vi "oa_Full Spectrum Transform (Spectra).vi"(6 "direction":u16(ring)=1 items=["CCW", "CW"], 7 "shift reverse spectrum (T)":bool=TRUE, 9 "phase lag spectrum (X-Y)":cluster{"x0":dbl, "dx":dbl, "phase":dbl[]}, 10 "Y magnitude spectrum":cluster{"x0":dbl, "dx":dbl, "magnitude":dbl[]}, 11 "X magnitude spectrum":cluster{"x0":dbl, "dx":dbl, "magnitude":dbl[]}) -> (2 "reverse precession spectrum":cluster{"x0":dbl, "dx":dbl, "magnitude":dbl[]}, 3 "forward precession spectrum":cluster{"x0":dbl, "dx":dbl, "magnitude":dbl[]})   [LabVIEW 2017]
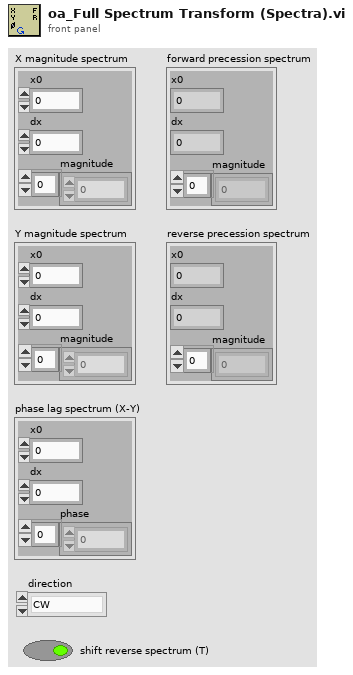
[diagram p1: front panel]
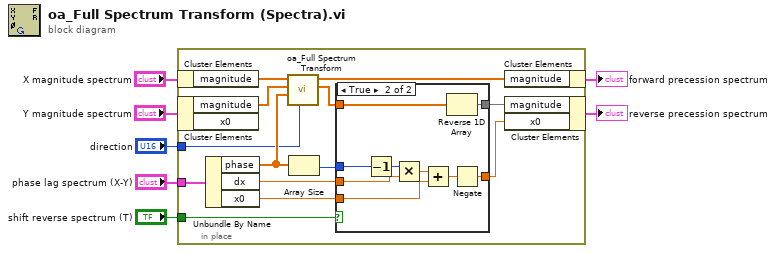
[diagram p0: block diagram]
diagram:
  n1 = in-place {
    in-place-border: "phase lag spectrum (X-Y)" -> [w17]
    in-place-border: "direction" -> [w16]
    in-place-border: "shift reverse spectrum (T)" -> [w8]
    n2 = in-place-cluster #1("X magnitude spectrum") -> ("magnitude"=w13:dbl[])
    n3 = in-place-cluster #2("Y magnitude spectrum") -> ("magnitude"=w14:dbl[])  [unwired: 1 out]
    n4 = Unbundle By Name(w17) -> ("phase"=w20:dbl[], "dx"=w18:dbl, "x0"=w19:dbl)
    n5 = call <vilib>:"oa_Full Spectrum Transform.vi"("direction"=w16, "Phase Lag (X-Y in radians)"=w20, "Y Magnitude"=w14, "X Magnitude"=w13) -> ("Reverse Precession Magnitude"=w10:dbl[], "Forward Precession Magnitude"=w12:dbl[])  [unwired: 6 in]
    n6 = Array Size(array=w20) -> (size(s)=w15:i32)
    n7 = case shown="True" w8 {
      tunnel: w19 -> [w21 w31]
      tunnel: w18 -> [_ w30]
      tunnel: w15 -> [_ w26]
      tunnel: [w21 w25] -> w11
      tunnel: w10 -> [w22 w24]
      tunnel: [w22 w23] -> w9
      frame False {
      }
      frame True {
        n8 = Decrement(x=w26) -> (x-1=w27:i32)
        n9 = Multiply(x=w27, y=w30) -> (x*y=w28:dbl)
        n10 = Add(x=w28, y=w31) -> (x+y=w29:dbl)
        n11 = Reverse 1D Array(array=w24) -> (reversed array=w23:dbl[])
        n12 = Negate(x=w29) -> (-x=w25:dbl)
      }
    }
    n13 = in-place-cluster #1("magnitude"=w12) -> (→"forward precession spectrum":cluster{"x0":dbl, "dx":dbl, "magnitude":dbl[]})
    n14 = in-place-cluster #2("magnitude"=w9, "x0"=w11) -> (→"reverse precession spectrum":cluster{"x0":dbl, "dx":dbl, "magnitude":dbl[]})
  }
